vi "Test View Stop Sent to View if Cleared while Running.vi"(8 "error in (no error)":errorcluster, 11 "View Test In":refnum<class "View Dev Test.lvclass">) -> (0 "error out":errorcluster, 3 "View Test Out":refnum<class "View Dev Test.lvclass">)   [LabVIEW 2020, in "View Dev Test.lvclass"]
uses:
  View Dev Test.lvclass
  C:/Program Files (x86)/National Instruments/LabVIEW 2020/vi.lib/Astemes/LUnit/Test Case.lvclass
  source/Framework/Process/Process.lvclass/Process.ctl
  <vilib>/Astemes/LUnit/Test Case.lvclass/Test Case.ctl
  <vilib>/Astemes/LUnit/LUnit Assertion Result.lvclass/LUnit Assertion Result.ctl
  <vilib>/Astemes/LUnit/LUnit Test Case Result.lvclass/LUnit Test Case Result.ctl
  <vilib>/Astemes/LUnit/LUnit Method Result.lvclass/LUnit Method Result.ctl
  source/Framework/Process/Public/Lifecycle/Get Lifecycle State.vi
  source/Framework/Broadcast Event Helpers/Execution timer.vi
  <vilib>/Astemes/LUnit/Set Assertion Type.vi
  <vilib>/Astemes/LUnit/Palette/Pass.vi
  <vilib>/Astemes/LUnit/Palette/Fail.vi
  <vilib>/Utility/error.llb/Clear Errors.vi
  <vilib>/Astemes/LUnit/LUnit Write Assertion Type.vi
  <vilib>/Astemes/LUnit/Add test result.vi
  <vilib>/Astemes/LUnit/LUnit Write Passed.vi
  <vilib>/Astemes/LUnit/LUnit Write Message.vi
  <vilib>/Astemes/LUnit/LUnit Write Description.vi
  <vilib>/Astemes/LUnit/LUnit Record Assertion Result.vi
  <vilib>/Astemes/LUnit/LUnit Aggregate Assertion Results.vi
  <vilib>/Astemes/LUnit/Assertion Result/LUnit Read Status.vi
  <vilib>/Astemes/LUnit/LUnit Read Message.vi
  <vilib>/Astemes/LUnit/LUnit Read Description.vi
  <vilib>/Astemes/LUnit/Method Result/LUnit Merge Status.vi
  <vilib>/Astemes/LUnit/LUnit Concatenate result strings.vi
  source/Framework/View/View.lvclass
  C:/Git/astemes-triarc-framework/source/Framework/Process/Process.lvclass
  <vilib>/Utility/error.llb/Error Cluster From Error Code.vi
  source/Framework/Broadcast Event Helpers/Dequeue Broadcast Message.vi
  <vilib>/Astemes/LUnit/LUnit Assertion Result.lvclass
  source/Framework/Process/Process.lvclass
  source/Framework/Broadcast Event Helpers/Broadcast Event Helpers.lvlib
  <vilib>/Astemes/LUnit/Test Case.lvclass
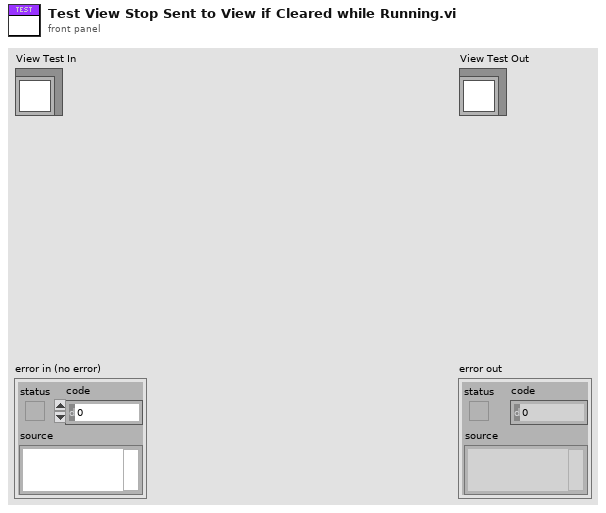
[diagram p1: front panel]
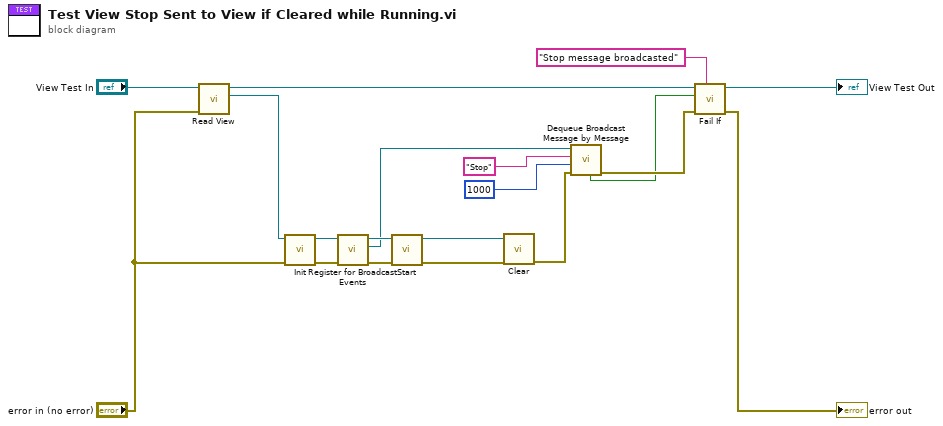
[diagram p0: block diagram]
diagram:
  n1 = call "Read View.vi"("error in (no error)"="error in (no error)", "View Test In"="View Test In") -> ("View"=w19:refnum<class "View.lvclass">, "View Test Out"=w4:refnum<class "View Dev Test.lvclass">)  [unwired: 7 in, 1 out]
  n2 = call-dynamic "Init.vi"("error in (no error)"="error in (no error)", "View In"=w19) -> ("error out"=w16:errorcluster, "View Out"=w12:refnum<class "View.lvclass">)  [unwired: 8 in]
  n3 = call "Register for Broadcast Events.vi"("error in (no error)"=w16, "Process In"=w12) -> ("error out"=w13:errorcluster, "Event Registration Refnum Out"=w10:refnum<event-registration>, "Process Out"=w11:refnum<class "View.lvclass">)  [unwired: 7 in]
  n4 = call "Start.vi"("error in (no error)"=w13, "Process In"=w11) -> ("error out"=w14:errorcluster, "Process Out"=w15:refnum<class "View.lvclass">)  [unwired: 7 in, 1 out]
  n5 = call-dynamic "Clear.vi"("error in (no error)"=w14, "View In"=w15) -> ("error out"=w9:errorcluster)  [unwired: 9 in]
  n6 = call "Dequeue Broadcast Message by Message.vi"("error in (no error)"=w9, "Timeout (-1)"=1000, "Message"="Stop", "Event Registration Refnum"=w10) -> ("error out"=w8:errorcluster, "Timed Out?"=w2:bool)  [unwired: 3 in, 3 out]
  n7 = call <vilib>:"Fail If.vi"("Description"="Stop message broadcasted", "error in (no error)"=w8, "Fail?"=w2, "LUnit Test Case In"=w4) -> ("error out"=→"error out":errorcluster, "LUnit Test Case Out"=→"View Test Out":refnum<class "View Dev Test.lvclass">)  [unwired: 6 in]
